vi "HapticSPM_force_only.vi"() -> ()   [LabVIEW 2023]
uses:
  Haptic-Programming-Interface/LabVIEW VIs/Haptic Prog Interface/Haptic Prog Interface.lvlib
  Haptic-Programming-Interface/src/x64/Debug/Haptic Programming Interface.dll
panel:
  out "Force Function":string
  in  "Input Function":i32 min=0 max=2 step=1
  out "Potential vs Distance":cluster{dbl[], dbl[]}(graph)
  out "Force vs Distance":cluster{dbl[], dbl[]}(graph)
  in  "Suggested Settings":bool=TRUE
  out "Z-Position":dbl caption="Numeric" format="%#.17p"
  out "Force":dbl(knob) scale=-3.0..3.0
  in  "k":dbl=1.0 caption="Numeric" step=0.1 format="%.1g"
  in  "Setpoint":dbl=1e-10 caption="Numeric" step=1e-11 format="%.0p"
  in  "Gain":dbl=1.0 caption="Numeric" format="%.1g"
  # "Super Ultra Mega Haptic SPM Controller 3000"
  # "Signal"
  # "Height"
  # "Move pen in all three dimensions to calibrate before feeling surface\n\nClick \"ENTER\" to turn off recommended settings\n\nChange \"Setpoint\" and \"k\" parameters to adjust the feel of the force\n\nUse the \"PAGE UP\" or \"PAGE DOWN\" key to change the force function"
  # "Force"
  # "Force"
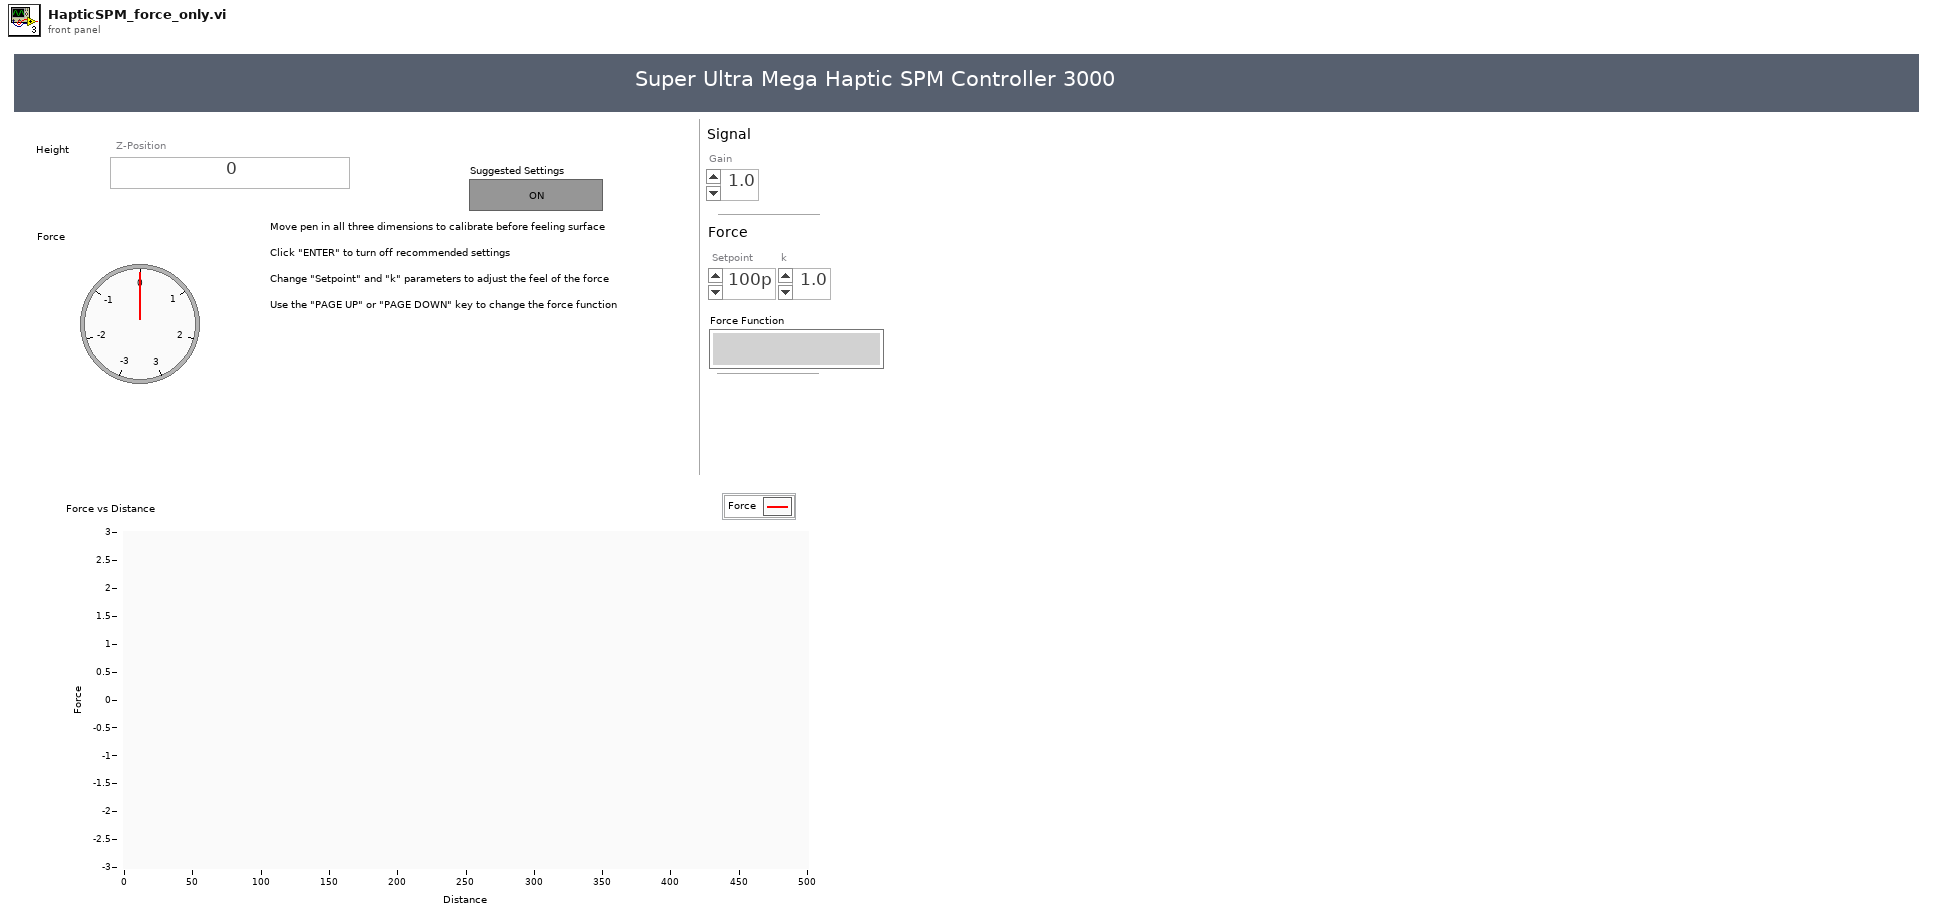
[diagram p1: front panel]
types:
  T1 = cluster{"Fx (N)":dbl, "Fy (N)":dbl, "Fz (N)":dbl}
  T2 = cluster{"kx (N/m)":dbl, "ky (N/m)":dbl, "kz (N/m)":dbl}
  T3 = cluster{"X Drag":bool, "Y Drag":bool, "Z Drag":bool}
  T4 = cluster{"x (mm)":dbl, "y (mm)":dbl, "z (mm)":dbl}
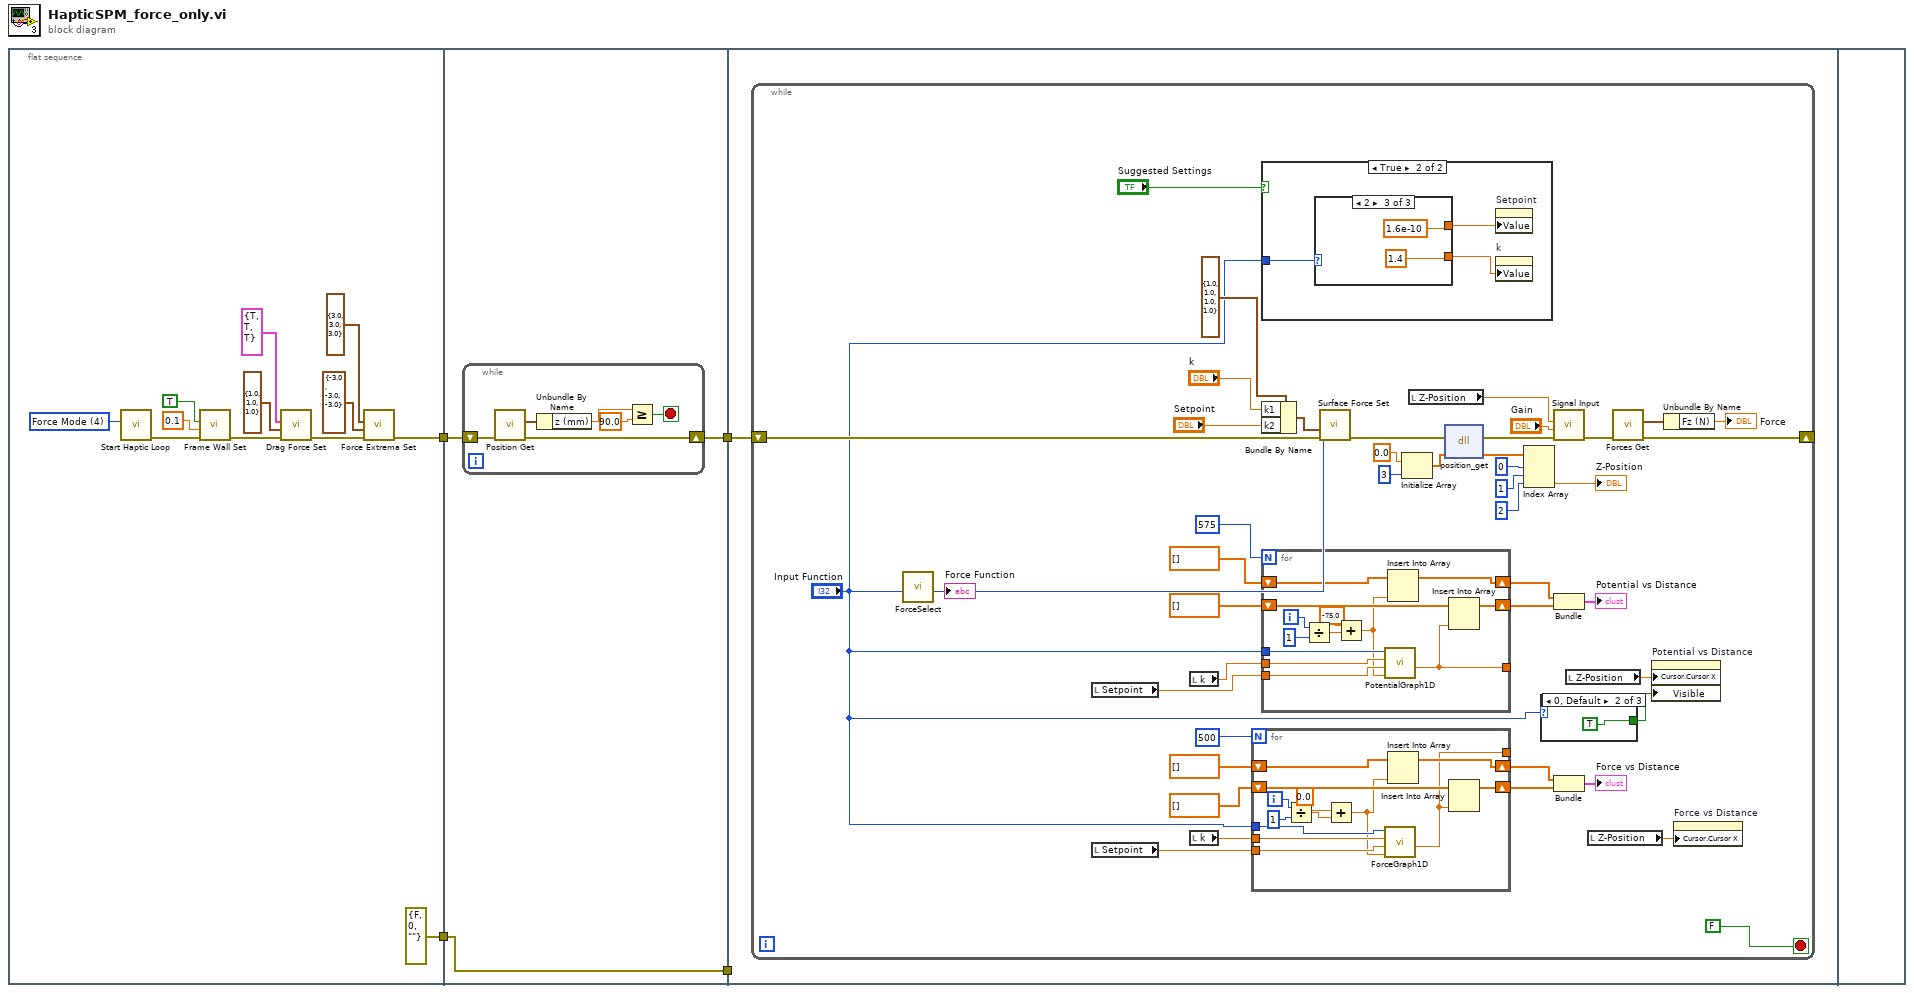
[diagram p0: block diagram]
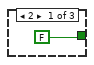
[diagram p2: hidden frame]
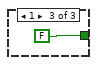
[diagram p3: hidden frame]
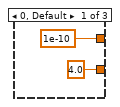
[diagram p5: hidden frame]
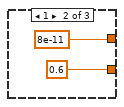
[diagram p6: hidden frame]
diagram:
  n1 = flat-sequence {
    tunnel: [w14] -> w4
    tunnel: [errorcluster {"status"=FALSE, "code"=0, "source"=""} ("error out")] -> w1
    tunnel: w4 -> [w19]
    tunnel: [w18] -> w3
    tunnel: [w17] -> w2
    tunnel: w1 -> [w17]
    tunnel: w3 -> [w26]
    tunnel: w2 -> [_]
    frame #0 {
      w16 = u16 4 items=["Custom Mode", "Read Mode", "Write Mode", "Virtual Mode", "Force Mode"] ("Mode Selection")
      n2 = call "Start Haptic Loop.vi"("Mode Selection"=w16) -> ("error out"=w7:errorcluster)  [unwired: 10 in]
      n3 = call "Frame Wall Set.vi"("error in (no error)"=w7, "Wall Stiffness (N/m)"=0.1 ("Wall Stiffness"), "Restrict to Frame"=TRUE) -> ("error out"=w6:errorcluster)  [unwired: 8 in]
      n4 = call "Drag Force Set.vi"("error in (no error)"=w6, "Drag Coefficients (N/m)"=T2 {"kx (N/m)"=1.0, "ky (N/m)"=1.0, "kz (N/m)"=1.0} ("Drag Coefficients"), "Drag Force Toggles"=T3 {"X Drag"=TRUE, "Y Drag"=TRUE, "Z Drag"=TRUE}) -> ("error out"=w15:errorcluster)  [unwired: 8 in]
      n5 = call "Force Extrema Set.vi"("error in (no error)"=w15, "Minimum Force (N)"=T1 {"Fx (N)"=-3.0, "Fy (N)"=-3.0, "Fz (N)"=-3.0} ("Minimum Force"), "Maximum Force (N)"=T1 {"Fx (N)"=3.0, "Fy (N)"=3.0, "Fz (N)"=3.0} ("Maximum Force")) -> ("error out"=w14:errorcluster)  [unwired: 8 in]
    }
    frame #1 {
      n6 = while {
        shift-right: [w24] -> w18
        shift-left: w19 -> [w25]
        stop <- w20 stop-if-true
        n7 = call "Position Get.vi"("error in (no error)"=w25) -> ("error out"=w24:errorcluster, "Position"=w23:T4)  [unwired: 9 in]
        n8 = Unbundle By Name(w23) -> ("z (mm)"=w22:dbl)
        n9 = Greater Or Equal?(x=w22, y=90.0) -> (x >= y?=w20:bool)
      }
    }
    frame #2 {
      n10 = while {
        shift-right: [w41] -> _
        shift-left: w26 -> [w70]
        stop <- FALSE ("Boolean") stop-if-true
        n11 = call "ForceSelect.vi"("Input Function"="Input Function") -> ("Force Function"=→"Force Function":string)  [unwired: 10 in]
        n12 = local read "Setpoint"() -> (w31:dbl)
        n13 = local read "Setpoint"() -> (w52:dbl)
        n14 = local read "k"() -> (w32:dbl)
        n15 = local read "k"() -> (w53:dbl)
        n16 = for {
          N: 500 -> [_]
          shift-right: [w99] -> w58
          shift-left: dbl[] [] -> [w97]
          shift-right: [w98] -> w59
          shift-left: dbl[] [] -> [w96]
          tunnel: "Input Function" -> [w92]
          tunnel: [w95] -> _
          tunnel: w52 -> [w94]
          tunnel: w53 -> [w93]
          i -> [w90]
          n17 = Divide(x=w90, y=1) -> (x/y=w89:dbl)
          n18 = Add(x=0.0, y=w89) -> (x+y=w87:dbl)
          n19 = call "ForceGraph1D.vi"("number"=w87, "Setpoint"=w94, "k"=w93, "Function"=w92) -> ("force"=w95:dbl)  [unwired: 7 in]
          n20 = Insert Into Array(array=w96, new element=w87) -> (w98:dbl[])  [unwired: 1 in]
          n21 = Insert Into Array(array=w97, new element=w95) -> (w99:dbl[])  [unwired: 1 in]
        }
        n22 = case shown="True" "Suggested Settings" {
          tunnel: "Input Function" -> [_ w102]
          frame False {
          }
          frame True {
            n23 = case shown="2" w102 {
              tunnel: [4.0 0.6 1.4] -> w101
              tunnel: [1e-10 8e-11 1.6e-10] -> w100
              frame 0, Default {
              }
              frame 1 {
              }
              frame 2 {
              }
            }
            n24 = property on="Setpoint" class="DigNum (strict)"("Value"=w100) -> ()  [unwired: 2 in, 2 out]
            n25 = property on="k" class="DigNum (strict)"("Value"=w101) -> ()  [unwired: 2 in, 2 out]
          }
        }
        n26 = Bundle By Name(cluster=cluster{"k1":dbl, "k2":dbl, "k3":dbl, "k4":dbl} {"k1"=1.0, "k2"=1.0, "k3"=1.0, "k4"=1.0} ("Force Constants"), "k1"="k", "k2"="Setpoint") -> (w66:cluster{"k1":dbl, "k2":dbl, "k3":dbl, "k4":dbl})
        n27 = for {
          N: 575 -> [_]
          shift-right: [w86] -> w37
          shift-left: dbl[] [] -> [w84]
          shift-right: [w85] -> w38
          shift-left: dbl[] [] -> [w83]
          tunnel: "Input Function" -> [w79]
          tunnel: [w82] -> _
          tunnel: w31 -> [w81]
          tunnel: w32 -> [w80]
          i -> [w77]
          n28 = Divide(x=w77, y=1) -> (x/y=w76:dbl)
          n29 = Add(x=-75.0, y=w76) -> (x+y=w74:dbl)
          n30 = call "PotentialGraph1D.vi"("number"=w74, "Setpoint"=w81, "k"=w80, "Function"=w79) -> ("potential"=w82:dbl)  [unwired: 7 in]
          n31 = Insert Into Array(array=w83, new element=w74) -> (w85:dbl[])  [unwired: 1 in]
          n32 = Insert Into Array(array=w84, new element=w82) -> (w86:dbl[])  [unwired: 1 in]
        }
        n33 = call "Surface Force Set.vi"("error in (no error)"=w70, "Force Constants"=w66, "Force Settings"="Input Function") -> ("error out"=w47:errorcluster)  [unwired: 8 in]
        n34 = Initialize Array(0.0 ("element"), 3 ("dimension size")) -> (w48:dbl[])
        n35 = local read "Z-Position"() -> (w63:dbl)
        n36 = dll-call lib="C:/Users/cjwel/Documents/GitHub/Haptic-Programming-Interface/src/x64/Debug/Haptic Programming Interface.dll" fn="position_get"(error in=w47, "output"=w48) -> (error out=w46:errorcluster, "output"=w42:dbl[])  [unwired: 3 in, 1 out]
        n37 = Index Array(array=w42, index #1=0 ("index"), index #2=1 ("index"), index #3=2 ("index")) -> (element #3=→"Z-Position":dbl)  [unwired: 2 out]
        n38 = case shown="0, Default" "Input Function" {
          tunnel: [FALSE TRUE FALSE] -> w29
          frame 2 {
          }
          frame 0, Default {
          }
          frame 1 {
          }
        }
        n39 = call "Signal Input.vi"("error in (no error)"=w46, "Gain"="Gain", "Signal"=w63) -> ("error out"=w69:errorcluster)  [unwired: 8 in]
        n40 = Bundle(w38, w37) -> (→"Potential vs Distance":cluster{dbl[], dbl[]})  [unwired: 1 in]
        n41 = Bundle(w59, w58) -> (→"Force vs Distance":cluster{dbl[], dbl[]})  [unwired: 1 in]
        n42 = local read "Z-Position"() -> (w30:dbl)
        n43 = local read "Z-Position"() -> (w51:dbl)
        n44 = call "Forces Get.vi"("error in (no error)"=w69) -> ("error out"=w41:errorcluster, "Force (N)"=w62:T1)  [unwired: 9 in]
        n45 = property on="Potential vs Distance" class="XYGraph (strict)"("Cursor.Cursor X"=w30, "Visible"=w29) -> ()  [unwired: 2 in, 2 out]
        n46 = Unbundle By Name(w62) -> ("Fz (N)"=→"Force":dbl)
        n47 = property on="Force vs Distance" class="XYGraph (strict)"("Cursor.Cursor X"=w51) -> ()  [unwired: 2 in, 2 out]
      }
    }
    frame #3 {
    }
  }
